vi "Main.vi"(8 "error in (no error)":errorcluster, 11 "Process in":refnum<class "STS Process.lvclass">) -> (0 "error out":errorcluster, 3 "Process out":refnum<class "STS Process.lvclass">)   [LabVIEW 2019, in "TimingDRV Engine.lvlib" / "STS Process.lvclass"]
uses:
  STS Process.lvclass
  C:/Users/XEnderMD/Desktop/CD Project Tools/Source/Engine/Parent Classes/Process/Process.lvclass
  STS Process.lvclass/STS Process.ctl
  Parent Classes/Process/Process.lvclass
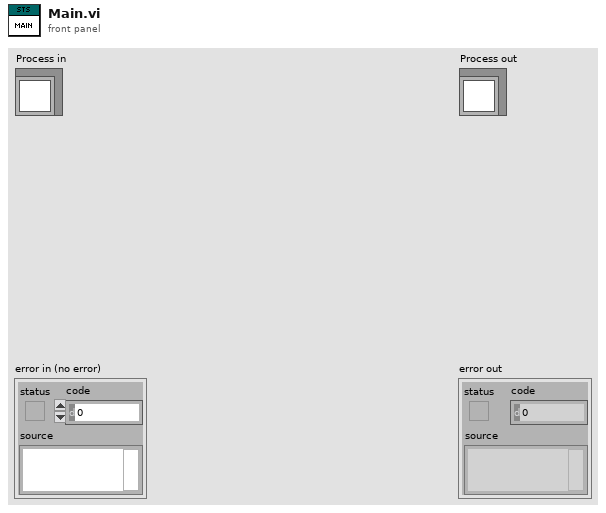
[diagram p1: front panel]
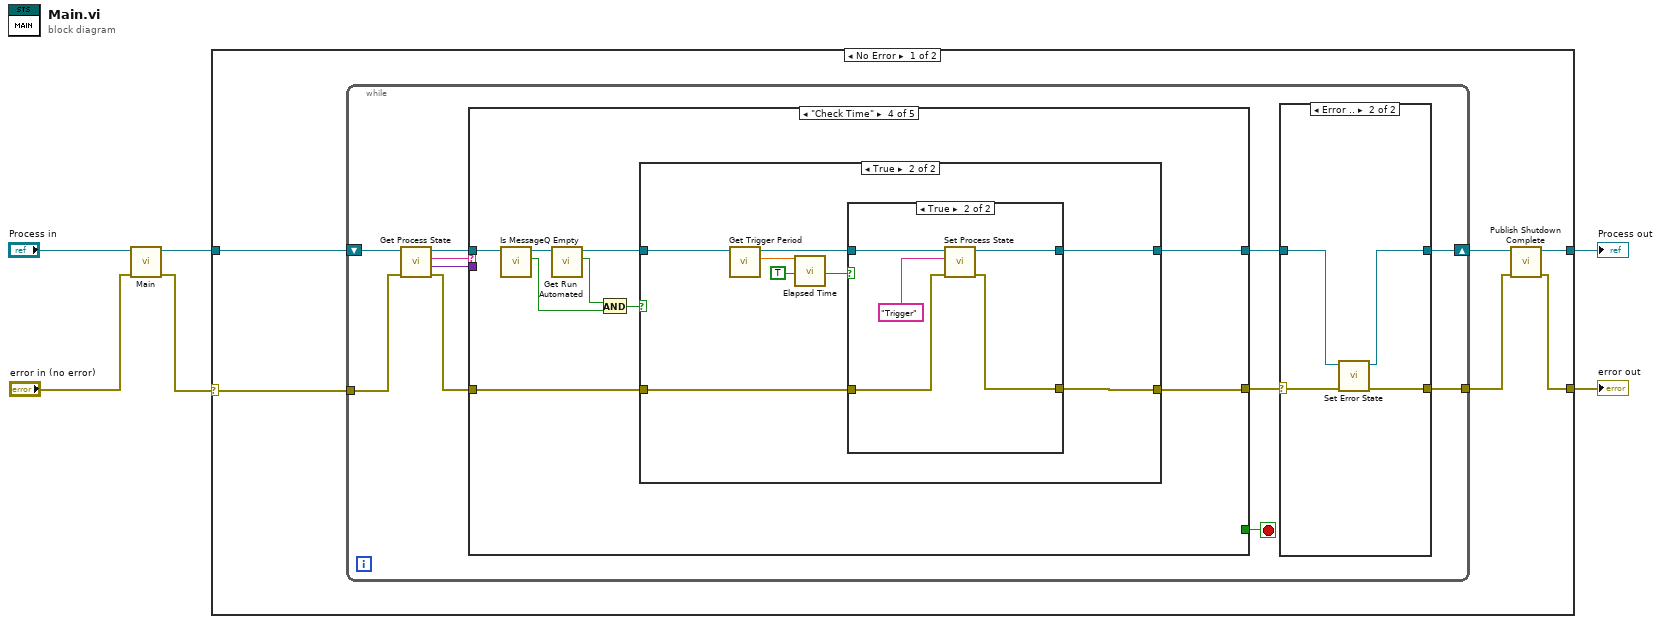
[diagram p0: block diagram]
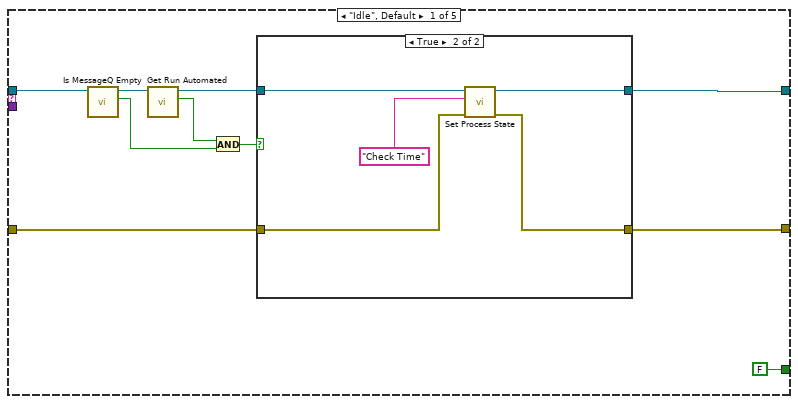
[diagram p3: hidden frame]
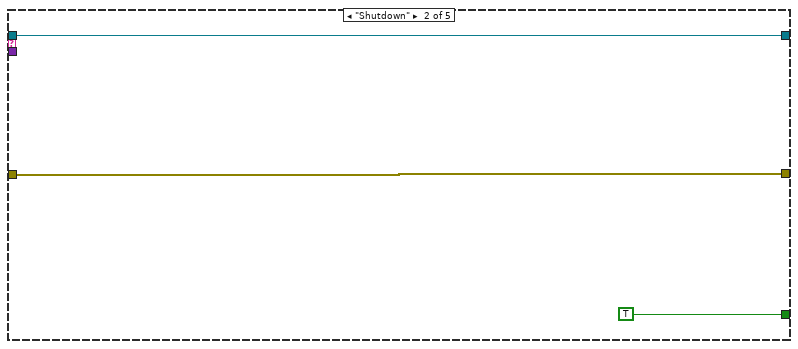
[diagram p5: hidden frame]
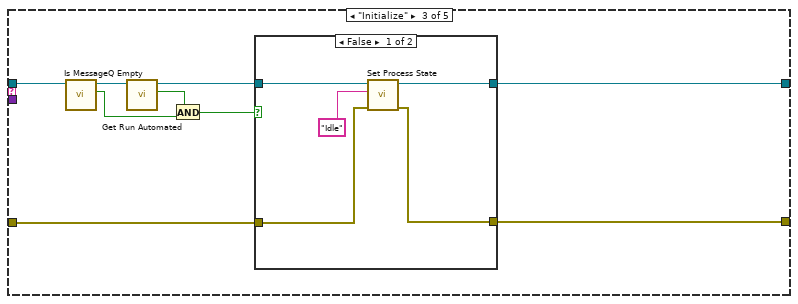
[diagram p6: hidden frame]
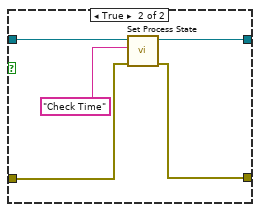
[diagram p7: hidden frame]
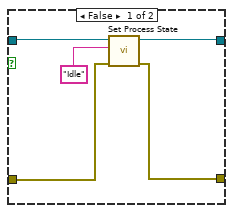
[diagram p9: hidden frame]
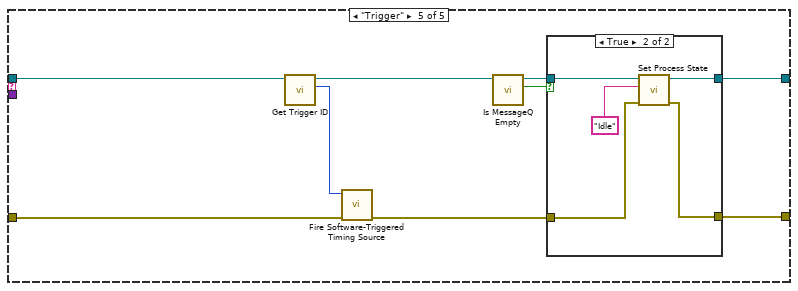
[diagram p10: hidden frame]
diagram:
  n1 = call-parent "Main.vi"("error in (no error)"="error in (no error)", "Process in"="Process in") -> ("error out"=w3:errorcluster, "Process out"=w4:refnum<class "STS Process.lvclass">)  [unwired: 8 in]
  n2 = case shown="No Error" w3 {
    selector: w3 -> [w8 w115]
    tunnel: [w9 w115] -> w1
    tunnel: [w11 w114] -> w2
    tunnel: w4 -> [w7 w114]
    frame No Error {
      n3 = while {
        shift-right: [w15] -> w12
        shift-left: w7 -> [w22]
        tunnel: w8 -> [w23]
        tunnel: [w14] -> w10
        stop <- w13 stop-if-true
        n4 = call "Get Process State.vi"("error in (no error)"=w23, "Process in"=w22) -> ("error out"=w18:errorcluster, "Payload"=w19:variant, "Command"=w20:string, "Process out"=w21:refnum<class "STS Process.lvclass">)  [unwired: 6 in]
        n5 = case shown="\"Check Time\"" w20 {
          tunnel: w21 -> [w36 w48 w54 w73 w105]
          tunnel: w19 -> [_ _ _ _ _]
          tunnel: w18 -> [w34 w47 w58 w76 w104]
          tunnel: [w38 w48 w57 w74 w98] -> w17
          tunnel: [w37 w47 w56 w75 w99] -> w16
          tunnel: [FALSE TRUE _ _ _] -> w13
          frame "Idle", Default {
            n6 = call "Is MessageQ Empty.vi"("Process in"=w36) -> ("is Empty ?"=w31:bool, "Process out"=w35:refnum<class "STS Process.lvclass">)  [unwired: 8 in, 1 out]
            n7 = call "Get Run Automated.vi"("STS Process in"=w35) -> ("Run Automated"=w32:bool, "STS Process out"=w33:refnum<class "STS Process.lvclass">)  [unwired: 9 in]
            n8 = And(x=w32, y=w31) -> (x .and. y?=w30:bool)
            n9 = case shown="True" w30 {
              tunnel: w33 -> [w41 w46]
              tunnel: [w41 w44] -> w38
              tunnel: w34 -> [w40 w43]
              tunnel: [w40 w42] -> w37
              frame False {
              }
              frame True {
                n10 = call "Set Process State.vi"("error in (no error)"=w43, "Command"="Check Time", "Process in"=w46) -> ("error out"=w42:errorcluster, "Process out"=w44:refnum<class "STS Process.lvclass">)  [unwired: 7 in]
              }
            }
          }
          frame "Shutdown" {
          }
          frame "Initialize" {
            n11 = call "Is MessageQ Empty.vi"("Process in"=w54) -> ("is Empty ?"=w51:bool, "Process out"=w53:refnum<class "STS Process.lvclass">)  [unwired: 8 in, 1 out]
            n12 = call "Get Run Automated.vi"("STS Process in"=w53) -> ("Run Automated"=w52:bool, "STS Process out"=w55:refnum<class "STS Process.lvclass">)  [unwired: 9 in]
            n13 = And(x=w52, y=w51) -> (x .and. y?=w50:bool)
            n14 = case shown="False" w50 {
              tunnel: w58 -> [w60 w68]
              tunnel: [w61 w67] -> w57
              tunnel: [w59 w66] -> w56
              tunnel: w55 -> [w62 w64]
              frame False {
                n15 = call "Set Process State.vi"("error in (no error)"=w60, "Command"="Idle", "Process in"=w62) -> ("error out"=w59:errorcluster, "Process out"=w61:refnum<class "STS Process.lvclass">)  [unwired: 7 in]
              }
              frame True {
                n16 = call "Set Process State.vi"("error in (no error)"=w68, "Command"="Check Time", "Process in"=w64) -> ("error out"=w66:errorcluster, "Process out"=w67:refnum<class "STS Process.lvclass">)  [unwired: 7 in]
              }
            }
          }
          frame "Check Time" {
            n17 = call "Is MessageQ Empty.vi"("Process in"=w73) -> ("is Empty ?"=w70:bool, "Process out"=w72:refnum<class "STS Process.lvclass">)  [unwired: 8 in, 1 out]
            n18 = call "Get Run Automated.vi"("STS Process in"=w72) -> ("Run Automated"=w71:bool, "STS Process out"=w77:refnum<class "STS Process.lvclass">)  [unwired: 9 in]
            n19 = And(x=w71, y=w70) -> (x .and. y?=w69:bool)
            n20 = case shown="True" w69 {
              tunnel: w77 -> [w79 w87]
              tunnel: w76 -> [w78 w82]
              tunnel: [w78 w81] -> w75
              tunnel: [w79 w80] -> w74
              frame False {
              }
              frame True {
                n21 = call "Get Trigger Period.vi"("STS Process in"=w87) -> ("Trigger Period"=w86:dbl, "STS Process out"=w83:refnum<class "STS Process.lvclass">)  [unwired: 9 in]
                n22 = call "Elapsed Time"("Time Target (s)"=w86, "Auto Reset"=TRUE) -> ("Time has Elapsed"=w84:bool)  [unwired: 10 in, 7 out]
                n23 = case shown="True" w84 {
                  tunnel: w83 -> [w91 w96]
                  tunnel: w82 -> [w90 w95]
                  tunnel: [w89 w94] -> w81
                  tunnel: [w88 w93] -> w80
                  frame False {
                    n24 = call "Set Process State.vi"("error in (no error)"=w90, "Command"="Idle", "Process in"=w91) -> ("error out"=w89:errorcluster, "Process out"=w88:refnum<class "STS Process.lvclass">)  [unwired: 7 in]
                  }
                  frame True {
                    n25 = call "Set Process State.vi"("error in (no error)"=w95, "Command"="Trigger", "Process in"=w96) -> ("error out"=w94:errorcluster, "Process out"=w93:refnum<class "STS Process.lvclass">)  [unwired: 7 in]
                  }
                }
              }
            }
          }
          frame "Trigger" {
            n26 = call "Get Trigger ID.vi"("STS Process in"=w105) -> ("Trigger ID"=w106:u8, "STS Process out"=w103:refnum<class "STS Process.lvclass">)  [unwired: 9 in]
            n27 = call <vilib>:"Fire Software-Triggered Timing Source.vi"("error in (no error)"=w104, "trigger ID"=w106) -> ("error out"=w100:errorcluster)  [unwired: 8 in, 1 out]
            n28 = call "Is MessageQ Empty.vi"("Process in"=w103) -> ("is Empty ?"=w102:bool, "Process out"=w101:refnum<class "STS Process.lvclass">)  [unwired: 8 in, 1 out]
            n29 = case shown="True" w102 {
              tunnel: w101 -> [w108 w112]
              tunnel: w100 -> [w107 w111]
              tunnel: [w107 w110] -> w99
              tunnel: [w108 w109] -> w98
              frame False {
              }
              frame True {
                n30 = call "Set Process State.vi"("error in (no error)"=w111, "Command"="Idle", "Process in"=w112) -> ("error out"=w110:errorcluster, "Process out"=w109:refnum<class "STS Process.lvclass">)  [unwired: 7 in]
              }
            }
          }
        }
        n31 = case shown="Error .." w16 {
          selector: w16 -> [w24 w29]
          tunnel: w17 -> [w25 w28]
          tunnel: [w25 w27] -> w15
          tunnel: [w24 w26] -> w14
          frame No Error {
          }
          frame Error {
            n32 = call "Set Error State.vi"("error in (no error)"=w29, "Process in"=w28) -> ("error out"=w26:errorcluster, "Process out"=w27:refnum<class "STS Process.lvclass">)  [unwired: 8 in]
          }
        }
      }
      n33 = call "Publish Shutdown Complete.vi"("error in (no error)"=w10, "Process in"=w12) -> ("error out"=w9:errorcluster, "Process out"=w11:refnum<class "STS Process.lvclass">)  [unwired: 8 in]
    }
    frame Error {
    }
  }
  "error out" <- w1
  "Process out" <- w2
